vi "BM0211-Image Editing.vi"(8 "error IN":errorcluster) -> (0 "error out":errorcluster)   [LabVIEW 2015]
uses:
  <vilib>/Utility/miscctls.llb/LVBoundsTypeDef.ctl
  <vilib>/Utility/miscctls.llb/LVPointTypeDef.ctl
panel:
  out "Assembly ST-1":picture
  out "filenames":string[](array[string])
  out "selected path":path
  out "Boolean":bool
  in  "Vertical position":sgl(slide) min=-2000 max=2000 scale=-1000.0..2000.0 scale format="%#.0f"
  in  "Horizontal position":sgl(slide) min=-2000 max=2000 scale=-1000.0..2000.0 scale format="%#.0f"
  in  "Zoom Factor":sgl(slide)=1.0 min=1 max=500 scale=0.0..500.0 scale format="%#.0f"
  out "2D Picture":picture
  in  "Stop Button":bool
  in  "Select Part":u16(ring) items=["P1.jpg", "P2.jpg", "P3.jpg", "P4.jpg", "P5.jpg", "P6.jpg", "P7.jpg", "P8.jpg", "P9.jpg", "P10.jpg", "P11.jpg", "P12.jpg", "P13.jpg", "P14.jpg", "P15.jpg", "P16.jpg", "P17.jpg", "P18.jpg"]
  in  "Save":bool
  in  "Select New":bool
  # "Image Editing"
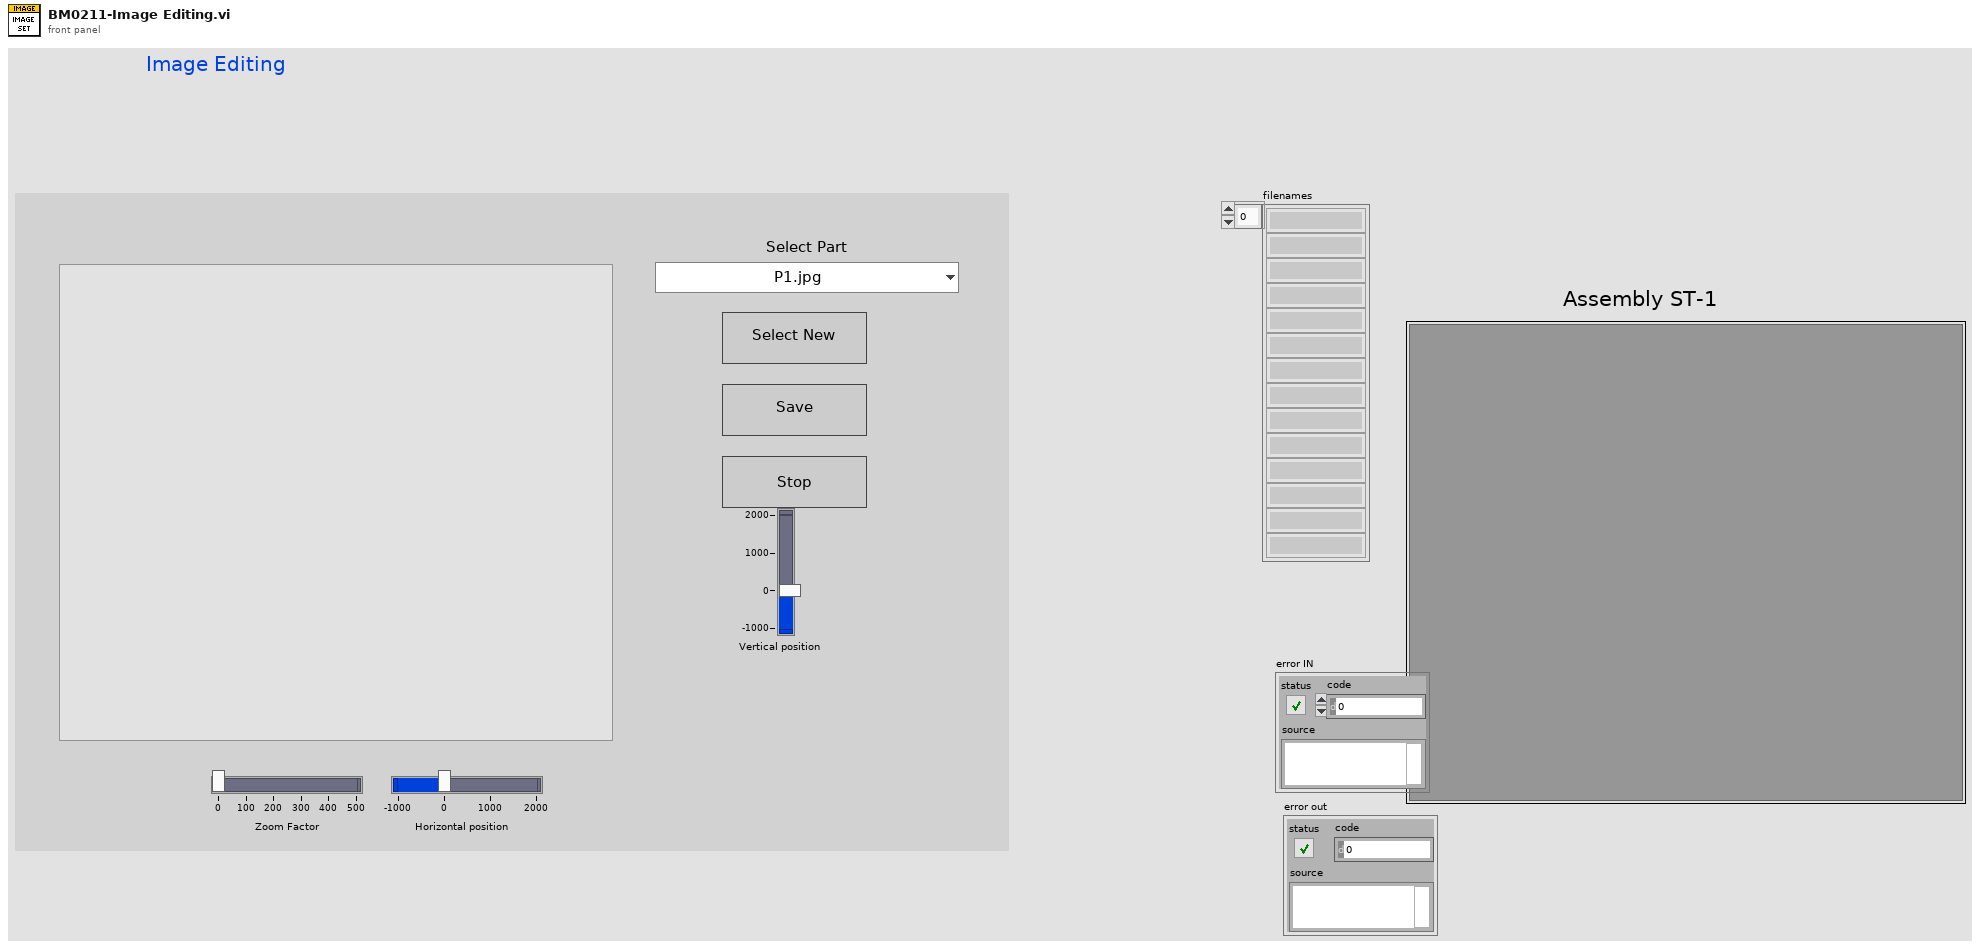
[diagram p1: front panel]
types:
  T1 = typedef "imagedata.ctl" = cluster{"image type":i32, "image depth":i32, "image":u8[], "mask":u8[], "colors":u32[], "Rectangle":cluster{"left":i16, "top":i16, "right":i16, "bottom":i16}}
  T2 = cluster{"Zoom Factor":sgl, "Horizontal position":sgl, "Vertical position":sgl}[]
  T3 = cluster{"Zoom Factor":sgl, "Horizontal position":sgl, "Vertical position":sgl}
  T4 = typedef "LVPointTypeDef.ctl" = cluster{"Horizontal":i16, "Vertical":i16}
  T5 = typedef "LVBoundsTypeDef.ctl" = cluster{"Width":u32, "Height":u32}
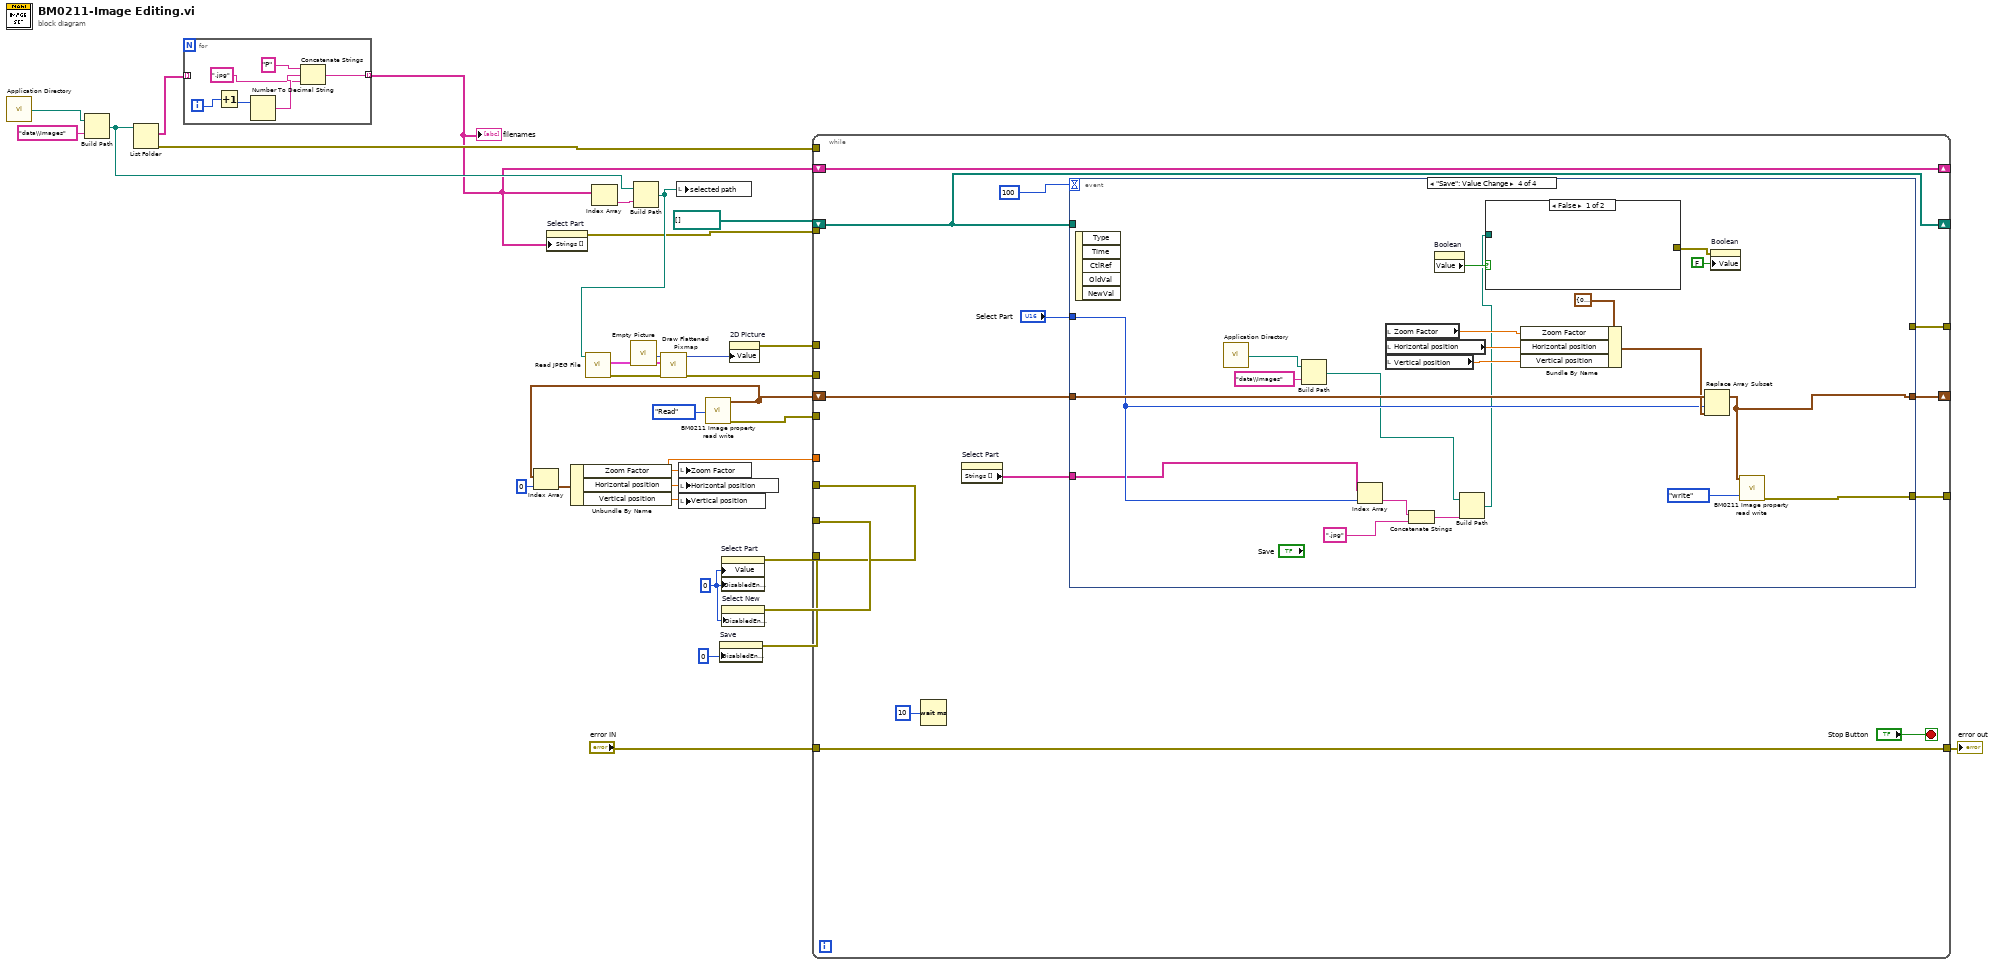
[diagram p0: block diagram]
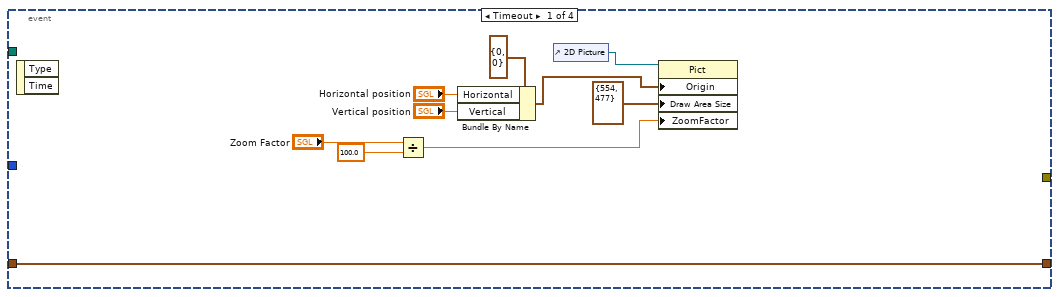
[diagram p2: hidden frame]
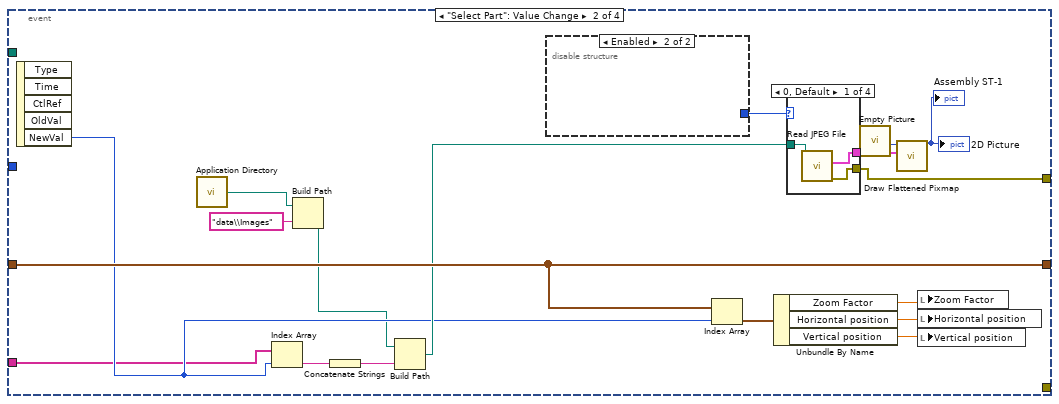
[diagram p3: hidden frame]
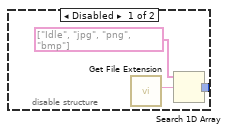
[diagram p4: hidden frame]
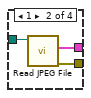
[diagram p5: hidden frame]
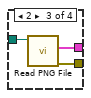
[diagram p6: hidden frame]
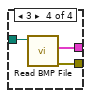
[diagram p7: hidden frame]
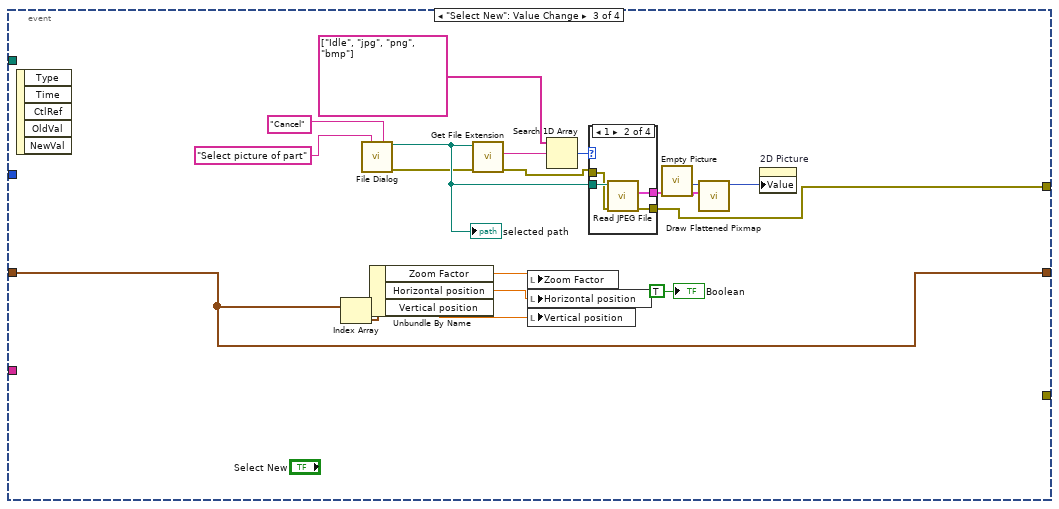
[diagram p8: hidden frame]
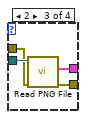
[diagram p10: hidden frame]
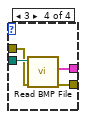
[diagram p11: hidden frame]
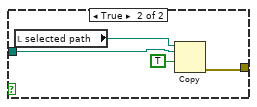
[diagram p12: hidden frame]
diagram:
  w14 = 0
  n1 = call <vilib>:"Application Directory.vi"() -> ("Application Directory"=w8:path)
  n2 = Build Path(base path=w8, name or relative path="data\\Images") -> (appended path=w6:path)
  n3 = List Folder(path=w6) -> (filenames=w2:string[], error out=w13:errorcluster)  [unwired: 3 in, 2 out]
  n4 = for {
    tunnel: w2 -> [_] mode=indexing
    tunnel: [w31] -> w1 mode=indexing
    i -> [w35]
    n5 = Increment(x=w35) -> (x+1=w36:i32)
    n6 = Number To Decimal String(number=w36) -> (decimal integer string=w34:string)  [unwired: 1 in]
    n7 = Concatenate Strings("P" ("string"), w34, ".jpg") -> (w31:string)
  }
  "filenames" <- w1
  n8 = property on="Select Part" class="Ring (strict)"("Strings []"=w1) -> (error out=w5:errorcluster)  [unwired: 2 in, 1 out]
  n9 = Index Array(array=w1) -> (element=w12:string)  [unwired: 1 in]
  n10 = call "Empty Picture"() -> ("empty picture"=w20:picture)
  n11 = Build Path(base path=w6, name or relative path=w12) -> (appended path=w9:path)
  n12 = call <vilib>:"Read JPEG File.vi"("path to JPEG file"=w9) -> ("error out"=w18:errorcluster, "image data"=w19:T1)  [unwired: 8 in, 1 out]
  n13 = call <vilib>:"Draw Flattened Pixmap.vi"("image data"=w19, "picture"=w20) -> ("new picture"=w17:picture)  [unwired: 7 in]
  n14 = local write "selected path"(w9) -> ()
  n15 = call "BM0211 Image property read write.vi"("Read write"=enum16{"write", "Read"}."Read") -> ("error out"=w10:errorcluster, "Out"=w23:T2)  [unwired: 9 in]
  n16 = Index Array(array=w23, index=0) -> (element=w24:T3)
  n17 = Unbundle By Name(w24) -> ("Zoom Factor"=w21:sgl, "Horizontal position"=w25:sgl, "Vertical position"=w26:sgl)
  n18 = local write "Zoom Factor"(w21) -> ()
  n19 = local write "Horizontal position"(w25) -> ()
  n20 = local write "Vertical position"(w26) -> ()
  n21 = property on="Save" class="Bool"("DisabledEnum"=0) -> (error out=w27:errorcluster)  [unwired: 2 in, 1 out]
  n22 = property on="Select Part" class="Ring (strict)"("Value"=w14, "DisabledEnum"=w14) -> (error out=w29:errorcluster)  [unwired: 2 in, 1 out]
  n23 = property on="Select New" class="Bool"("DisabledEnum"=w14) -> (error out=w30:errorcluster)  [unwired: 2 in, 1 out]
  n24 = property on="2D Picture" class="Pict"("Value"=w17) -> (error out=w16:errorcluster)  [unwired: 2 in, 1 out]
  n25 = while {
    shift-right: [w46] -> _
    shift-left: path[] [] ("Array") -> [w46]
    tunnel: [w45] -> _
    shift-right: [w42] -> _
    shift-left: w23 -> [w44]
    tunnel: w30 -> [_]
    tunnel: w29 -> [_]
    tunnel: w27 -> [_]
    tunnel: w21 -> [_]
    tunnel: w18 -> [_]
    tunnel: w16 -> [_]
    tunnel: w13 -> [_]
    shift-right: [w40] -> _
    shift-left: w1 -> [w40]
    tunnel: w10 -> [_]
    tunnel: [w39] -> _
    tunnel: w5 -> [_]
    tunnel: "error IN" -> [w37]
    tunnel: [w37] -> w3
    stop <- "Stop Button" stop-if-true
    n26 = Wait (ms)(milliseconds to wait=u32 10) -> ()  [unwired: 1 out]
    n27 = property on="Select Part" class="Ring (strict)"() -> ("Strings []"=w38:string[])  [unwired: 2 in, 2 out]
    n28 = event shown="[3] \"Save\": Value Change" {
      selector: _ -> [_ _ _ _]
      dyn-events: _ -> [_ _ _ _]
      timeout: 100 -> [_ _ _ _]
      tunnel: w46 -> [_ _ _ _]
      tunnel: [_ w75 w98 _] -> w45
      tunnel: w44 -> [w49 w72 w96 w136]
      tunnel: "Select Part" -> [_ _ _ w133]
      tunnel: [w49 w72 w96 w128] -> w42
      tunnel: [_ _ _ w131] -> w39
      tunnel: w38 -> [_ w60 _ w124]
      event Timeout {
        n29 = event-data() -> ()  [unwired: 1 in, 2 out]
        n30 = Divide(x="Zoom Factor", y=sgl 100.0 ("x")) -> (x/y=w55:sgl)
        n31 = Bundle By Name(cluster=T4 {"Horizontal"=0, "Vertical"=0} ("Origin"), "Horizontal"="Horizontal position", "Vertical"="Vertical position") -> (w51:T4)
        n32 = control-ref of="2D Picture"() -> (w56:refnum<vi>)
        n33 = property class="Pict"(reference=w56, "Origin"=w51, "Draw Area Size"=T5 {"Width"=554, "Height"=477}, "ZoomFactor"=w55) -> ()  [unwired: 1 in, 2 out]
      }
      event "Select Part": Value Change {
        n34 = event-data() -> ("NewVal"=w64:u16)  [unwired: 1 in, 4 out]
        n35 = call <vilib>:"Application Directory.vi"() -> ("Application Directory"=w63:path)
        n36 = Index Array(array=w60, index=w64) -> (element=w67:string)
        n37 = Build Path(base path=w63, name or relative path="data\\Images") -> (appended path=w61:path)
        n38 = Concatenate Strings(w67) -> (w65:string)
        n39 = Build Path(base path=w61, name or relative path=w65) -> (appended path=w66:path)
        n40 = disable-structure shown="Enabled" {
          disable-tunnel: [w77 _] -> w74
          frame Disabled {
            n41 = call <vilib>:"Get File Extension.vi"() -> ("lowercase file extension"=w78:string)  [unwired: 7 in, 4 out]
            n42 = Search 1D Array(1D array=string[] ["Idle", "jpg", "png", "bmp"] ("Strings []"), element=w78) -> (index of element=w77:i32)  [unwired: 1 in]
          }
          frame Enabled {
          }
        }
        n43 = Index Array(array=w72, index=w64) -> (element=w71:T3)
        n44 = Unbundle By Name(w71) -> ("Zoom Factor"=w70:sgl, "Horizontal position"=w69:sgl, "Vertical position"=w68:sgl)
        n45 = case shown="0, Default" w74 {
          tunnel: [w81 w85 w87 w90] -> w73
          tunnel: [w80 w84 w86 w91] -> w75
          tunnel: w66 -> [w82 w83 w88 w89]
          frame 0, Default {
            n46 = call <vilib>:"Read JPEG File.vi"("path to JPEG file"=w82) -> ("error out"=w80:errorcluster, "image data"=w81:T1)  [unwired: 8 in, 1 out]
          }
          frame 1 {
            n47 = call <vilib>:"Read JPEG File.vi"("path to JPEG file"=w83) -> ("error out"=w84:errorcluster, "image data"=w85:T1)  [unwired: 8 in, 1 out]
          }
          frame 2 {
            n48 = call <vilib>:"Read PNG File.vi"("path to PNG file"=w88) -> ("error out"=w86:errorcluster, "image data"=w87:T1)  [unwired: 8 in, 1 out]
          }
          frame 3 {
            n49 = call <vilib>:"Read BMP File.vi"("path to BMP file"=w89) -> ("error out"=w91:errorcluster, "image data"=w90:T1)  [unwired: 8 in, 1 out]
          }
        }
        n50 = call "Empty Picture"() -> ("empty picture"=w76:picture)
        n51 = call <vilib>:"Draw Flattened Pixmap.vi"("image data"=w73, "picture"=w76) -> ("new picture"=→"2D Picture" →"Assembly ST-1":picture)  [unwired: 7 in]
        n52 = local write "Zoom Factor"(w70) -> ()
        n53 = local write "Horizontal position"(w69) -> ()
        n54 = local write "Vertical position"(w68) -> ()
      }
      event "Select New": Value Change {
        n55 = event-data() -> ()  [unwired: 1 in, 5 out]
        n56 = Index Array(array=w96) -> (element=w95:T3)  [unwired: 1 in]
        n57 = call "File Dialog"("prompt"="Select picture of part", "button label"="Cancel") -> ("selected path"=w101:path, "error out"=w100:errorcluster)  [unwired: 10 in, 2 out]
        "selected path" <- w101
        n58 = Unbundle By Name(w95) -> ("Zoom Factor"=w94:sgl, "Horizontal position"=w93:sgl, "Vertical position"=w92:sgl)
        n59 = call <vilib>:"Get File Extension.vi"("error in (no error)"=w100, "file"=w101) -> ("error out"=w105:errorcluster, "lowercase file extension"=w107:string)  [unwired: 5 in, 3 out]
        n60 = local write "Zoom Factor"(w94) -> ()
        n61 = local write "Horizontal position"(w93) -> ()
        n62 = local write "Vertical position"(w92) -> ()
        n63 = Search 1D Array(1D array=string[] ["Idle", "jpg", "png", "bmp"] ("Strings []"), element=w107) -> (index of element=w106:i32)  [unwired: 1 in]
        n64 = case shown="1" w106 {
          tunnel: [_ w114 w118 w121] -> w99
          tunnel: [w110 w113 w117 w122] -> w98
          tunnel: w105 -> [w110 w111 w115 w119]
          tunnel: w101 -> [_ w112 w116 w120]
          frame 0, Default {
          }
          frame 1 {
            n65 = call <vilib>:"Read JPEG File.vi"("error in (no error)"=w111, "path to JPEG file"=w112) -> ("error out"=w113:errorcluster, "image data"=w114:T1)  [unwired: 7 in, 1 out]
          }
          frame 2 {
            n66 = call <vilib>:"Read PNG File.vi"("error in (no error)"=w115, "path to PNG file"=w116) -> ("error out"=w117:errorcluster, "image data"=w118:T1)  [unwired: 7 in, 1 out]
          }
          frame 3 {
            n67 = call <vilib>:"Read BMP File.vi"("error in (no error)"=w119, "path to BMP file"=w120) -> ("error out"=w122:errorcluster, "image data"=w121:T1)  [unwired: 7 in, 1 out]
          }
        }
        n68 = call "Empty Picture"() -> ("empty picture"=w109:picture)
        n69 = call <vilib>:"Draw Flattened Pixmap.vi"("image data"=w99, "picture"=w109) -> ("new picture"=w104:picture)  [unwired: 7 in]
        n70 = property on="2D Picture" class="Pict"("Value"=w104) -> ()  [unwired: 2 in, 2 out]
        "Boolean" <- TRUE
      }
      event "Save": Value Change {
        n71 = event-data() -> ()  [unwired: 1 in, 5 out]
        n72 = call <vilib>:"Application Directory.vi"() -> ("Application Directory"=w127:path)
        n73 = Build Path(base path=w127, name or relative path="data\\Images") -> (appended path=w125:path)
        n74 = Index Array(array=w124, index=w133) -> (element=w123:string)
        n75 = local read "Zoom Factor"() -> (w140:sgl)
        n76 = local read "Horizontal position"() -> (w139:sgl)
        n77 = local read "Vertical position"() -> (w138:sgl)
        n78 = Concatenate Strings(w123, ".jpg" ("string")) -> (w130:string)
        n79 = property on="Boolean" class="Bool (strict)"() -> ("Value"=w143:bool)  [unwired: 2 in, 2 out]
        n80 = Build Path(base path=w125, name or relative path=w130) -> (appended path=w132:path)
        n81 = case shown="False" w143 {
          tunnel: w132 -> [_ w144]
          tunnel: [_ w147] -> w141
          frame False {
          }
          frame True {
            n82 = local read "selected path"() -> (w146:path)
            n83 = Copy(9:TRUE ("overwrite (F)"), 10:w144, 11:w146) -> (0:w147:errorcluster)  [unwired: 2 in, 2 out]
          }
        }
        n84 = Bundle By Name(cluster=T3 {"Zoom Factor"=0.0, "Horizontal position"=0.0, "Vertical position"=0.0} ("element"), "Zoom Factor"=w140, "Horizontal position"=w139, "Vertical position"=w138) -> (w135:T3)
        n85 = Replace Array Subset(array=w136, new element=w135, index=w133) -> (w128:T2)
        n86 = property on="Boolean" class="Bool (strict)"(error in=w141, "Value"=FALSE ("Boolean")) -> ()  [unwired: 1 in, 2 out]
        n87 = call "BM0211 Image property read write.vi"("Read write"=enum16{"write", "Read"}."write", "IN"=w128) -> ("error out"=w131:errorcluster)  [unwired: 8 in, 1 out]
      }
    }
  }
  "error out" <- w3
